vi "Convert NT Cluster to Variant.vi"(11 "Field Value":T1) -> (3 "Variant":variant)   [LabVIEW 2017]
uses:
  <vilib>/Rock Robotics/Network Tables/Field Data.ctl
  <vilib>/Rock Robotics/Network Tables/Field Type.ctl
  <vilib>/Rock Robotics/Network Tables/Sequence.ctl
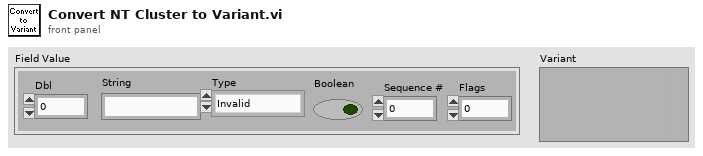
[diagram p1: front panel]
types:
  T1 = typedef "Field Data.ctl" = cluster{"Dbl":dbl, "String":string, "Type":T2, "Boolean":bool, "Sequence #":T3, "Flags":u8}
  T2 = typedef "Field Type.ctl" = enum8{"Invalid", "Bool", "Numeric", "String", "Raw", "Boolean Array", "Numeric Array", "String Array", "RPC"}
  T3 = typedef "Sequence.ctl" = u16
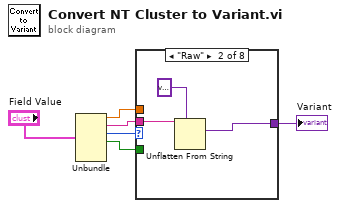
[diagram p0: block diagram]
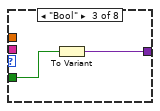
[diagram p3: hidden frame]
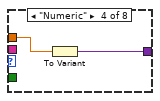
[diagram p4: hidden frame]
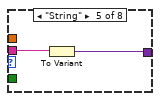
[diagram p5: hidden frame]
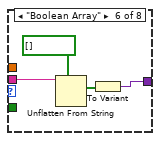
[diagram p6: hidden frame]
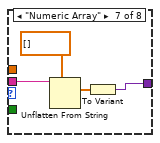
[diagram p7: hidden frame]
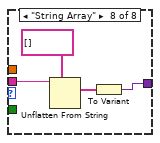
[diagram p8: hidden frame]
diagram:
  n1 = Unbundle("Field Value") -> ("Dbl"=w2:dbl, "String"=w3:string, "Type"=w5:T2, "Boolean"=w4:bool)  [unwired: 2 out]
  n2 = case shown="\"Raw\"" w5 {
    tunnel: w4 -> [_ _ w11 _ _ _ _ _]
    tunnel: w3 -> [_ w9 _ _ w15 w19 w20 w26]
    tunnel: w2 -> [_ _ _ w12 _ _ _ _]
    tunnel: [_ w8 w10 w13 w14 w17 w23 w24] -> w1
    frame "Invalid", Default {
    }
    frame "Raw" {
      n3 = Unflatten From String(type=variant, binary string=w9) -> (value=w8:variant)  [unwired: 3 in, 2 out]
    }
    frame "Bool" {
      n4 = To Variant(anything=w11) -> (Variant=w10:variant)
    }
    frame "Numeric" {
      n5 = To Variant(anything=w12) -> (Variant=w13:variant)
    }
    frame "String" {
      n6 = To Variant(anything=w15) -> (Variant=w14:variant)
    }
    frame "Boolean Array" {
      n7 = Unflatten From String(type=bool[] [], binary string=w19) -> (value=w16:bool[])  [unwired: 3 in, 2 out]
      n8 = To Variant(anything=w16) -> (Variant=w17:variant)
    }
    frame "Numeric Array" {
      n9 = Unflatten From String(type=dbl[] [], binary string=w20) -> (value=w22:dbl[])  [unwired: 3 in, 2 out]
      n10 = To Variant(anything=w22) -> (Variant=w23:variant)
    }
    frame "String Array" {
      n11 = Unflatten From String(type=string[] [], binary string=w26) -> (value=w25:string[])  [unwired: 3 in, 2 out]
      n12 = To Variant(anything=w25) -> (Variant=w24:variant)
    }
  }
  "Variant" <- w1
